vi "Decimate Data For 2D Intensity Chart - DVR.vi"(9 "Plot Area":T1, 11 "data value reference":refnum<data-value>) -> (3 "Decimated Display":u16[][](array[numeric]))   [LabVIEW 2026, in "MicroPulse_Driver.lvlib"]
uses:
  MicroPulse_Driver.lvlib
  <vilib>/Utility/miscctls.llb/LVBoundsTypeDef.ctl
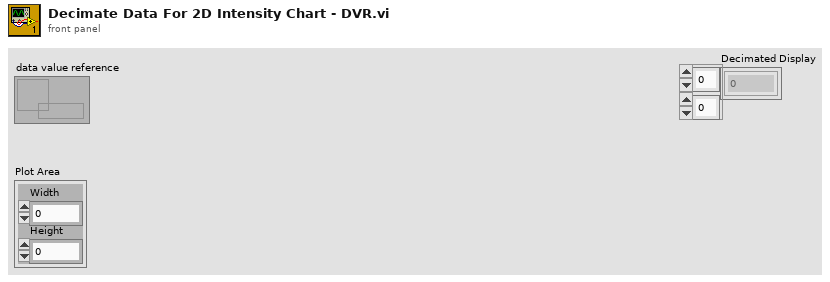
[diagram p1: front panel]
types:
  T1 = typedef "LVBoundsTypeDef.ctl" = cluster{"Width":u32, "Height":u32}
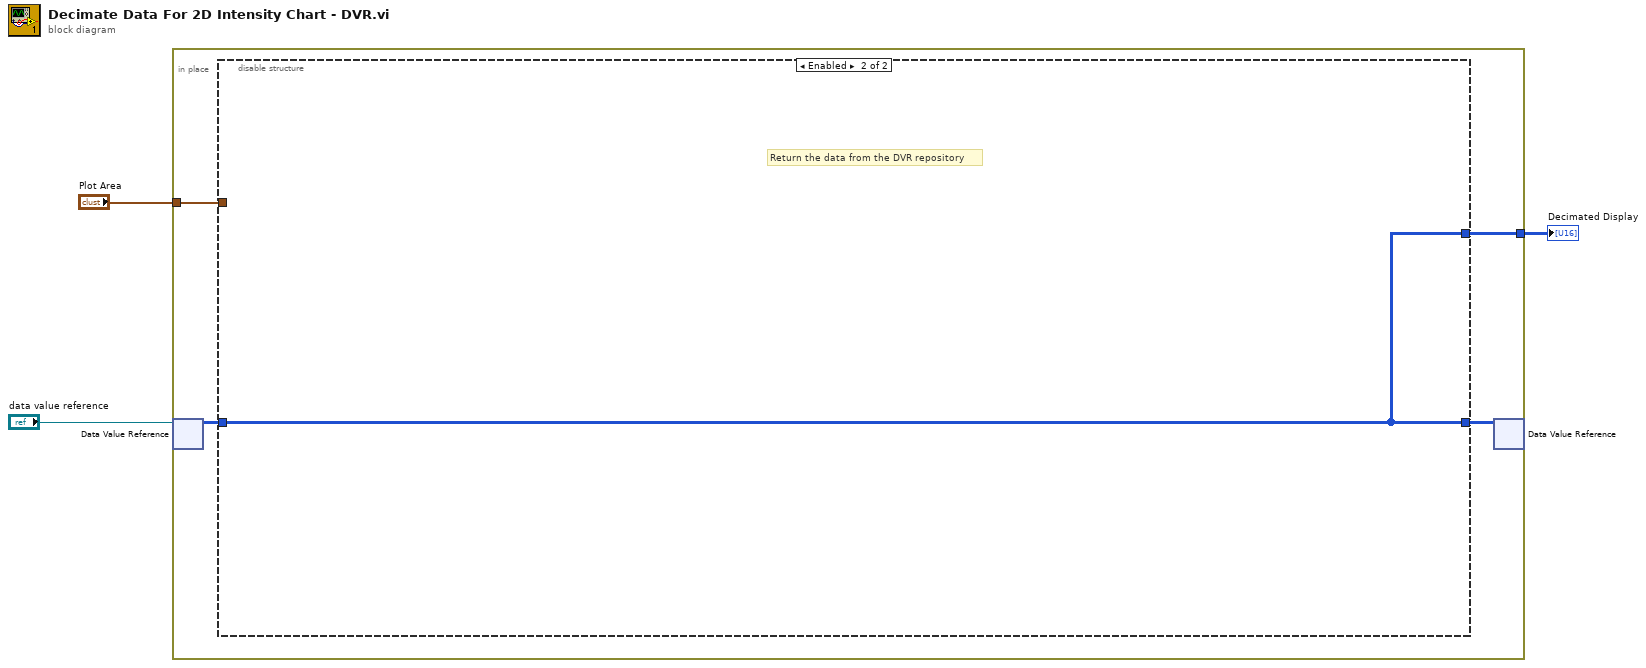
[diagram p0: block diagram]
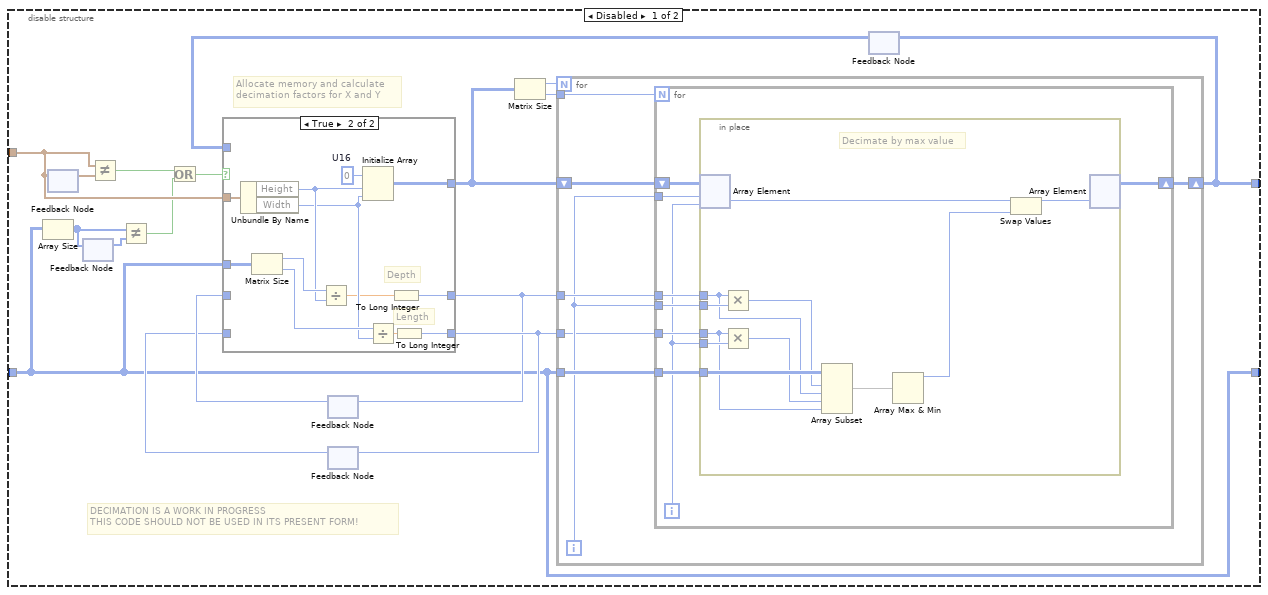
[diagram p2: hidden frame]
diagram:
  n1 = in-place {
    in-place-border: "Plot Area" -> [w7]
    in-place-border: [w6] -> w2
    n2 = in-place-dvr #1("data value reference") -> (w5:u16[][])  [unwired: 1 out]
    n3 = disable-structure shown="Enabled" {
      disable-tunnel: w7 -> [w22 _]
      disable-tunnel: [w21 w66] -> w6
      disable-tunnel: w5 -> [w8 w66]
      disable-tunnel: [w8 w66] -> w4
      frame Disabled {
        # "DECIMATION IS A WORK IN PROGRESS\nTHIS CODE SHOULD NOT BE USED IN ITS PRESENT FORM!"
        # "Allocate memory and calculate\ndecimation factors for X and Y"
        n4 = Array Size(array=w8) -> (size(s)=w12:i32[])
        n5 = feedback #2() -> (w24:T1)  [unwired: 1 in]
        n6 = feedback-in #2(w22) -> ()
        n7 = feedback #3() -> (w11:i32[])  [unwired: 1 in]
        n8 = feedback-in #3(w12) -> ()
        n9 = Not Equal?(x=w22, y=w24) -> (x != y?=w23:bool)
        n10 = Not Equal?(x=w12, y=w11) -> (x != y?=w9:bool)
        n11 = Or(x=w23, y=w9) -> (x .or. y?=w10:bool)
        n12 = feedback #4() -> (w19:i32)  [unwired: 1 in]
        n13 = feedback #5() -> (w17:i32)  [unwired: 1 in]
        n14 = feedback #6() -> (w20:u16[][])  [unwired: 1 in]
        n15 = case shown="True" w10 {
          tunnel: w22 -> [_ w39]
          tunnel: [w27 w37] -> w15
          tunnel: w20 -> [w27 _]
          tunnel: w8 -> [_ w36]
          tunnel: [w26 w29] -> w16
          tunnel: [w25 w28] -> w18
          tunnel: w19 -> [w26 _]
          tunnel: w17 -> [w25 _]
          frame False {
          }
          frame True {
            w38 = u16 0  # U16
            # "Length"
            # "Depth"
            n16 = Unbundle By Name(w39) -> ("Height"=w34:u32, "Width"=w32:u32)
            n17 = Matrix Size(0:w36) -> (1:w35:i32, 2:w33:i32)
            n18 = Divide(x=w35, y=w34) -> (x/y=w31:dbl)
            n19 = Initialize Array(w38, w34, w32) -> (w37:u16[][])
            n20 = Divide(x=w33, y=w32) -> (x/y=w30:dbl)
            n21 = To Long Integer(number=w31) -> (32bit integer=w29:i32)
            n22 = To Long Integer(number=w30) -> (32bit integer=w28:i32)
          }
        }
        n23 = feedback-in #4(w16) -> ()
        n24 = feedback-in #5(w18) -> ()
        n25 = Matrix Size(0:w15) -> (1:w14:i32, 2:w13:i32)
        n26 = for {
          N: w14 -> [_]
          shift-right: [w45] -> w21
          shift-left: w15 -> [w46]
          tunnel: w8 -> [w44]
          tunnel: w16 -> [w43]
          tunnel: w18 -> [w41]
          tunnel: w13 -> [w40]
          i -> [w42]
          n27 = for {
            N: w40 -> [_]
            shift-right: [w53] -> w45
            shift-left: w46 -> [w54]
            tunnel: w42 -> [w52]
            tunnel: w44 -> [w51]
            tunnel: w43 -> [w50]
            tunnel: w42 -> [w49]
            tunnel: w41 -> [w48]
            i -> [w47]
            n28 = in-place {
              in-place-border: w51 -> [w65]
              in-place-border: w50 -> [w60]
              in-place-border: w49 -> [w63]
              in-place-border: w48 -> [w59]
              in-place-border: w47 -> [w62]
              # "Decimate by max value"
              n29 = in-place-array #7(w54, w52, w47) -> (w57:u16)
              n30 = Multiply(x=w60, y=w63) -> (x*y=w64:i32)
              n31 = Multiply(x=w59, y=w62) -> (x*y=w61:i32)
              n32 = Array Subset(array=w65, index (row)=w64, length (row)=w60, index (col)=w61, length (col)=w59) -> (w58:u16[][])
              n33 = Array Max & Min(array=w58) -> (max value=w56:u16)  [unwired: 3 out]
              n34 = Swap Values(12:w57, 14:w56) -> (1:w55:u16)  [unwired: 1 in, 1 out]
              n35 = in-place-array #7(w55) -> (w53:u16[][])  [unwired: 2 out]
            }
          }
        }
        n36 = feedback-in #6(w21) -> ()
      }
      frame Enabled {
        # "Return the data from the DVR repository"
      }
    }
    n37 = in-place-dvr #1(w4) -> ()  [unwired: 2 out]
  }
  "Decimated Display" <- w2
